vi "thermo_var.vi"() -> ()   [LabVIEW 2020]
uses:
  thermo.ctl
  thermo_types.ctl
  Thermometer Fail Action.ctl
panel:
  in  "timeout":i32=5000 caption="Readout timeout [ms]" min=100 max=30000
  in  "retry N":i32=10 caption="Maximum readout tries" min=0 max=100
  in  "try fail":T1(ring)=enum."Stop trying - return zeroes" caption="Retries failed action"
  in  "channels":i32=2
  in  "last index":i32
  in  "thermos":T2[](array[typedef]) {"RTD inv" format="%.1f"; "RTD set" format="%.1f"; "temp cor" format="%.1f"; "RH cor" format="%.1f"; "pres cor" format="%.1f"; "refresh" min=0.1 max=1000.0 format="%.2f"}
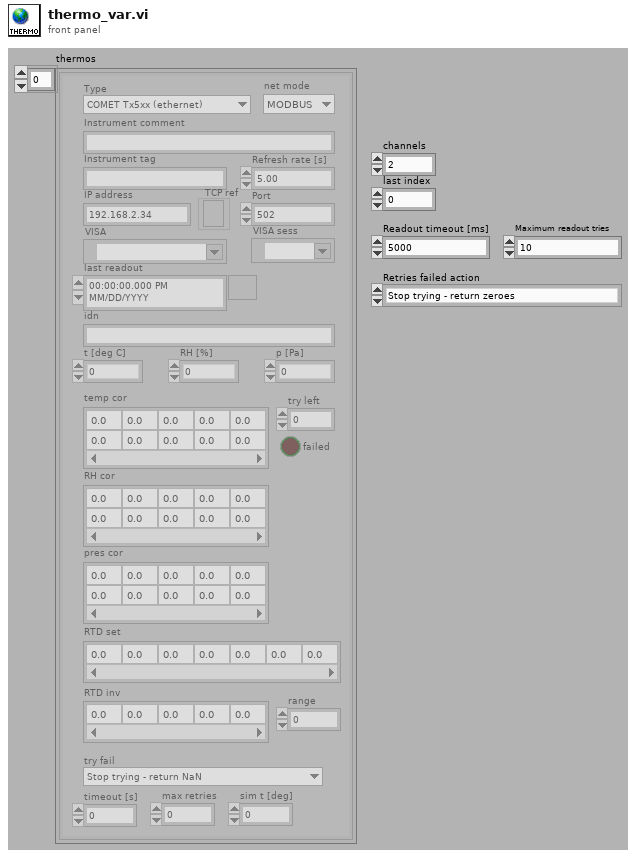
[diagram p1: front panel]
types:
  T1 = enum16{"Stop trying - keep last value", "Stop trying - return zeroes", "Generate error - stop sweep"}
  T2 = typedef "thermo.ctl" = cluster{"type":T3, "comment":string, "tag":string, "refresh":dbl, "IP":string, "port":u16, "VISA":refnum<visa-resource-name>, "last readout":timestamp, "TCP ref":refnum<k5>, "VISA sess":refnum<visa-resource-name>, "idn":string, "press":dbl, "RH":dbl, "temp":dbl, "pres cor":dbl[][], "RH cor":dbl[][], "temp cor":dbl[][], "try left":i32, "failed":bool, "RTD set":dbl[], "RTD inv":dbl[], "range":dbl, "net mode":enum16{"MODBUS", "HTTP"}, "try fail":T4, "timeout [s]":dbl, "max retries":i32, "sim t [deg]":dbl}
  T3 = typedef "thermo_types.ctl" = enum16{"Disabled", "Simulated", "COMET Tx5xx (ethernet)", "Keithley 2002 (GPIB) + RTD", "Agilent 344xx (GPIB) + RTD"}
  T4 = typedef "Thermometer Fail Action.ctl" = enum16{"Stop trying - keep last value", "Stop trying - return NaN", "Generate error - stop sweep"}
diagram:
